vi "_get_float.vi"(3 "错误输入（无错误）":errorcluster, 4 "写入缓冲区":string, 5 "连接ID":refnum<k5>) -> (0 "错误输出":errorcluster, 1 "数字":sgl, 2 "连接ID输出":refnum<k5>)   [LabVIEW 2017]
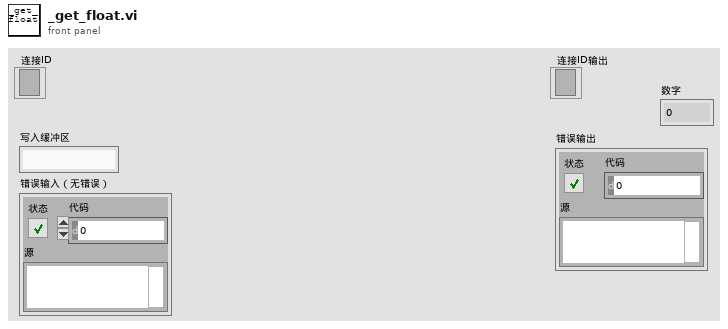
[diagram p1: front panel]
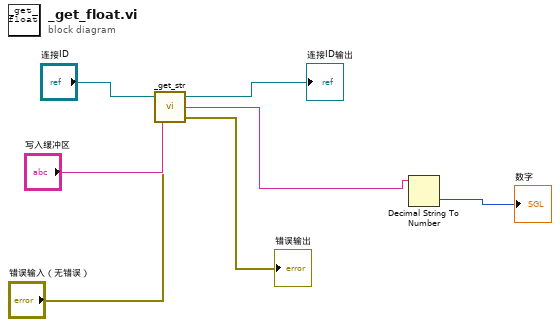
[diagram p0: block diagram]
diagram:
  n1 = call "_get_str.vi"("错误输入（无错误）"="错误输入（无错误）", "写入缓冲区"="写入缓冲区", "连接ID"="连接ID") -> ("错误输出"=→"错误输出":errorcluster, "读取缓冲区"=w4:string, "连接ID输出"=→"连接ID输出":refnum<k5>)
  n2 = Decimal String To Number(string=w4) -> (number=→"数字":i32)  [unwired: 2 in, 1 out]
